vi "USB2XXXIICAM2321.vi"() -> ()   [LabVIEW 2010]
panel:
  out "湿度/百分比":dbl
  out "温度/摄氏度":dbl
  out "湿度":dbl(slide) scale=0.0..100.0
  out "温度":dbl(slide) scale=0.0..100.0
  out "工作状态":bool
  in  "pConfig":T1
  in  "Channel Index":i32(ring) items=["CH0", "CH1", "CH2", "CH3", "CH4", "CH5", "CH6", "CH7"]
  in  "Device Index":i32(ring) items=["0", "1", "2", "3", "4", "5"]
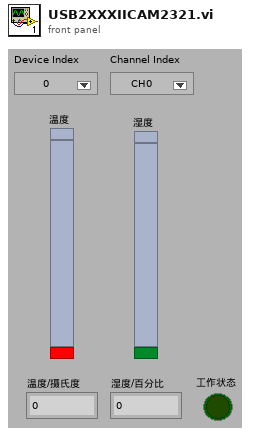
[diagram p1: front panel]
types:
  T1 = cluster{"ClockSpeedHz":u32, "OwnAddr":u16, "Master":u8, "AddrBits":u8, "EnablePu":u8}
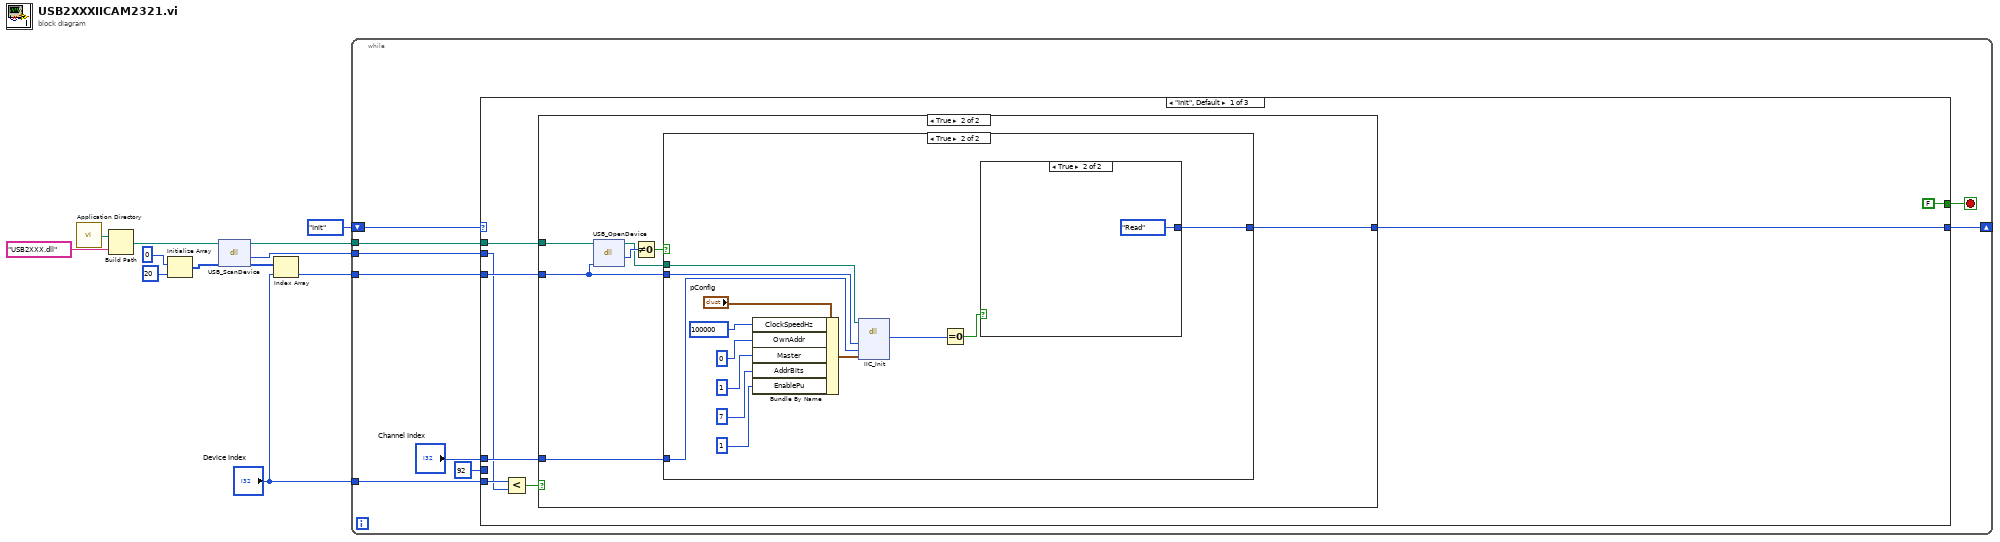
[diagram p0: block diagram]
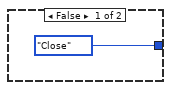
[diagram p2: hidden frame]
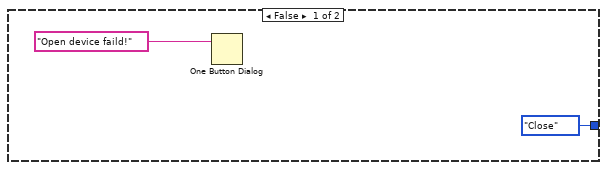
[diagram p3: hidden frame]
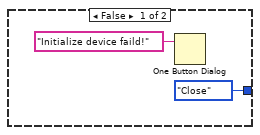
[diagram p4: hidden frame]
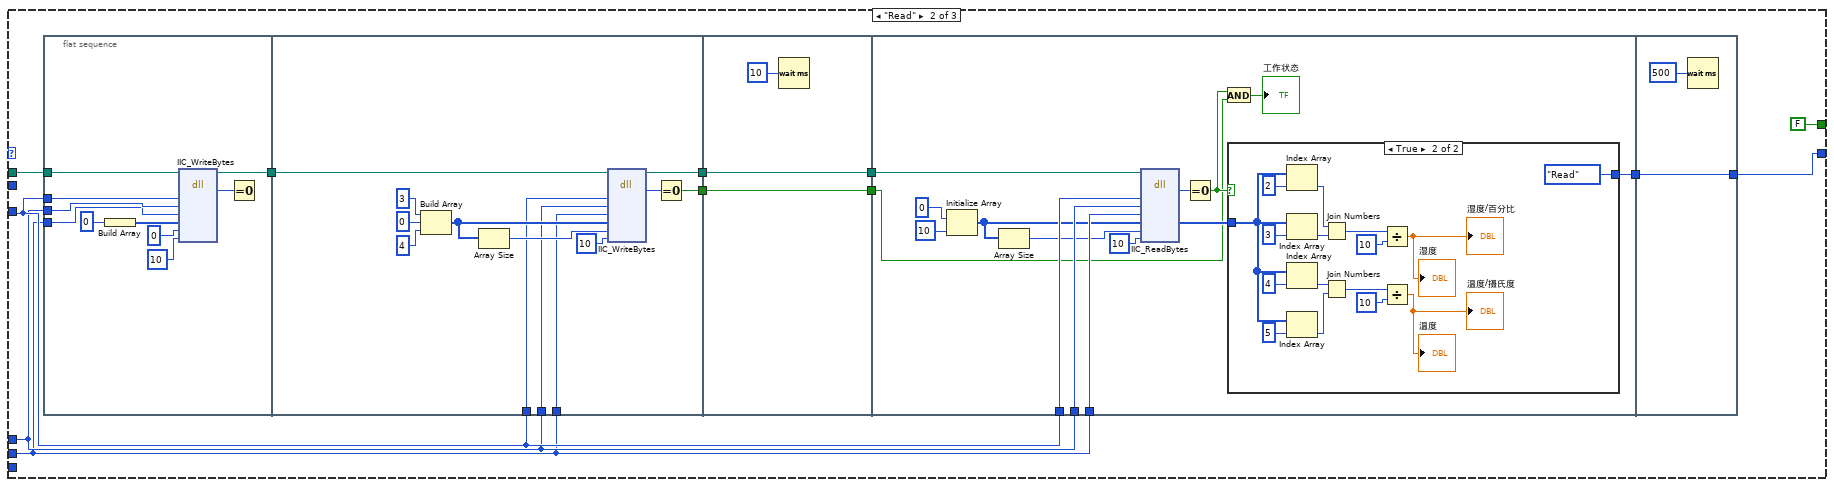
[diagram p5: hidden frame]
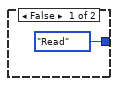
[diagram p6: hidden frame]
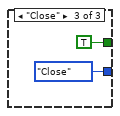
[diagram p7: hidden frame]
diagram:
  n1 = call <vilib>:"Application Directory.vi"() -> ("Application Directory"=w3:path)
  n2 = Build Path(base path=w3, name or relative path="USB2XXX.dll") -> (appended path=w2:path)
  n3 = Initialize Array(0, 20 ("dimension size")) -> (w8:i32[])
  n4 = dll-call lib="E:/Projects/USB2XXX_Example/sdk/api/Labview/USB2XXX.*" fn="USB_ScanDevice"(path in=w2, "pDevNum"=w8) -> (path out=w1:path, "return type"=w6:i32, "pDevNum"=w11:i32[])  [unwired: 2 in, 1 out]
  n5 = Index Array(array=w11, index="Device Index") -> (element=w7:i32)
  n6 = while {
    shift-right: [w20] -> _
    shift-left: enum16{"Init", "Read", "Close"}."Init" ("Enum") -> [w21]
    tunnel: w7 -> [w16]
    tunnel: w6 -> [w15]
    tunnel: "Device Index" -> [w14]
    tunnel: w1 -> [w13]
    stop <- w17 stop-if-true
    n7 = case shown="\"Init\", Default" w21 {
      tunnel: [w28 w63 enum16{"Init", "Read", "Close"}."Close" ("Enum")] -> w20
      tunnel: w16 -> [w27 w66 _]
      tunnel: "Channel Index" -> [w26 w65 _]
      tunnel: i16 92 ("Slave Addr(Hex)") -> [_ w64 _]
      tunnel: [FALSE FALSE TRUE] -> w17
      tunnel: w14 -> [w24 _ _]
      tunnel: w15 -> [w23 _ _]
      tunnel: w13 -> [w22 w59 _]
      frame "Init", Default {
        n8 = Less?(x=w24, y=w23) -> (x < y?=w29:bool)
        n9 = case shown="True" w29 {
          tunnel: w27 -> [_ w34]
          tunnel: w26 -> [_ w35]
          tunnel: [enum16{"Init", "Read", "Close"}."Close" ("Enum") w33] -> w28
          tunnel: w22 -> [_ w32]
          frame False {
          }
          frame True {
            n10 = dll-call lib="E:/Projects/USB2XXX_Example/sdk/api/Labview/USB2XXX.*" fn="USB_OpenDevice"(path in=w32, "DevIndex"=w34) -> (path out=w31:path, "return type"=w37:u8)  [unwired: 3 in, 1 out]
            n11 = Not Equal To 0?(x=w37) -> (x != 0?=w36:bool)
            n12 = case shown="True" w36 {
              tunnel: w35 -> [_ w44]
              tunnel: w34 -> [_ w45]
              tunnel: [enum16{"Init", "Read", "Close"}."Close" ("Enum") w41] -> w33
              tunnel: w31 -> [_ w40]
              frame False {
                n13 = One Button Dialog(message="Open device faild!") -> ()  [unwired: 1 in, 1 out]
              }
              frame True {
                n14 = Bundle By Name(cluster="pConfig", "ClockSpeedHz"=u32 100000, "OwnAddr"=u16 0, "Master"=u8 1, "AddrBits"=u8 7, "EnablePu"=u8 1) -> (w51:T1)
                n15 = dll-call lib="E:/Projects/USB2XXX_Example/sdk/api/Labview/USB2XXX.*" fn="IIC_Init"(path in=w40, "DevIndex"=w45, "IICIndex"=w44, "pConfig"=w51) -> ("return type"=w43:i32)  [unwired: 5 in, 2 out]
                n16 = Equal To 0?(x=w43) -> (x = 0?=w42:bool)
                n17 = case shown="True" w42 {
                  tunnel: [enum16{"Init", "Read", "Close"}."Close" ("Enum") enum16{"Init", "Read", "Close"}."Read" ("Enum")] -> w41
                  frame False {
                    n18 = One Button Dialog(message="Initialize device faild!") -> ()  [unwired: 1 in, 1 out]
                  }
                  frame True {
                  }
                }
              }
            }
          }
        }
      }
      frame "Read" {
        n19 = flat-sequence {
          tunnel: w66 -> [w74]
          tunnel: w65 -> [w73]
          tunnel: w64 -> [w72]
          tunnel: w59 -> [w69]
          tunnel: [w68] -> w58
          tunnel: w66 -> [w83]
          tunnel: w65 -> [w82]
          tunnel: w64 -> [w81]
          tunnel: [w80] -> w61
          tunnel: w58 -> [w79]
          tunnel: [w78] -> w56
          tunnel: w61 -> [w92]
          tunnel: [w92] -> w60
          tunnel: [w91] -> w57
          tunnel: w56 -> [w91]
          tunnel: w66 -> [w108]
          tunnel: w65 -> [w107]
          tunnel: w64 -> [w106]
          tunnel: [w98] -> w62
          tunnel: w60 -> [w95]
          tunnel: w57 -> [w94]
          tunnel: [w127] -> w63
          tunnel: w62 -> [w127]
          frame #0 {
            n20 = Build Array(u8 0 ("WriteLen")) -> (w71:u8[])
            n21 = dll-call lib="E:/Projects/USB2XXX_Example/sdk/api/Labview/USB2XXX.*" fn="IIC_WriteBytes"(path in=w69, "DevIndex"=w74, "IICIndex"=w73, "SlaveAddr"=w72, "pWriteData"=w71, "WriteLen"=0, "TimeOutMs"=10) -> (path out=w68:path, "return type"=w76:i32)  [unwired: 8 in, 1 out]
            n22 = Equal To 0?(x=w76) -> ()  [unwired: 1 out]
          }
          frame #1 {
            n23 = Build Array(u8 3, u8 0 ("element"), u8 4 ("element")) -> (w84:u8[])
            n24 = Array Size(array=w84) -> (size(s)=w90:i32)
            n25 = dll-call lib="E:/Projects/USB2XXX_Example/sdk/api/Labview/USB2XXX.*" fn="IIC_WriteBytes"(path in=w79, "DevIndex"=w83, "IICIndex"=w82, "SlaveAddr"=w81, "pWriteData"=w84, "WriteLen"=w90, "TimeOutMs"=10) -> (path out=w78:path, "return type"=w88:i32)  [unwired: 8 in, 1 out]
            n26 = Equal To 0?(x=w88) -> (x = 0?=w80:bool)
          }
          frame #2 {
            n27 = Wait (ms)(milliseconds to wait=u32 10) -> ()  [unwired: 1 out]
          }
          frame #3 {
            n28 = Initialize Array(u8 0 ("element"), 10 ("dimension size")) -> (w103:u8[])
            n29 = Array Size(array=w103) -> (size(s)=w102:i32)
            n30 = dll-call lib="E:/Projects/USB2XXX_Example/sdk/api/Labview/USB2XXX.*" fn="IIC_ReadBytes"(path in=w94, "DevIndex"=w108, "IICIndex"=w107, "SlaveAddr"=w106, "pReadData"=w103, "ReadLen"=w102, "TimeOutMs"=10) -> ("return type"=w100:i32, "pReadData"=w99:u8[])  [unwired: 7 in, 2 out]
            n31 = Equal To 0?(x=w100) -> (x = 0?=w96:bool)
            n32 = And(x=w96, y=w95) -> (x .and. y?=→"工作状态":bool)
            n33 = case shown="True" w96 {
              tunnel: w99 -> [_ w117]
              tunnel: [enum16{"Init", "Read", "Close"}."Read" ("Enum") enum16{"Init", "Read", "Close"}."Read" ("Enum")] -> w98
              frame False {
              }
              frame True {
                n34 = Index Array(array=w117, index=2) -> (element=w119:u8)
                n35 = Index Array(array=w117, index=3) -> (element=w118:u8)
                n36 = Index Array(array=w117, index=4) -> (element=w123:u8)
                n37 = Index Array(array=w117, index=5) -> (element=w122:u8)
                n38 = Join Numbers(hi=w119, lo=w118) -> ((hi.lo)=w116:u16)
                n39 = Join Numbers(hi=w123, lo=w122) -> ((hi.lo)=w114:u16)
                n40 = Divide(x=w116, y=u16 10) -> (x/y=→"湿度/百分比" →"湿度":dbl)
                n41 = Divide(x=w114, y=u16 10) -> (x/y=→"温度/摄氏度" →"温度":dbl)
              }
            }
          }
          frame #4 {
            n42 = Wait (ms)(milliseconds to wait=u32 500) -> ()  [unwired: 1 out]
          }
        }
      }
      frame "Close" {
      }
    }
  }
